vi "destroyDAQ.vi"(11 "handle":u32) -> (3 "Succés?":bool)   [LabVIEW 2020]
uses:
  cDaqlib/cDaq.lvlib
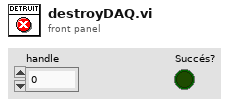
[diagram p1: front panel]
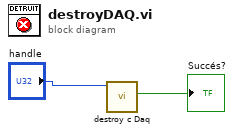
[diagram p0: block diagram]
diagram:
  n1 = call "destroy c Daq .vi"("handle"="handle") -> ("function return"=→"Succés?":bool)  [unwired: 9 in, 1 out]
